vi "Compute Residuals Absolute Area.vi"(8 "Error In":errorcluster, 11 "Residual Plot in":cluster{"X Array":dbl[], "Y Array":dbl[]}) -> (0 "Error Out":errorcluster, 2 "Residuals Area":dbl, 4 "Message":string)   [LabVIEW 2021, in "Fits.lvlib"]
uses:
  Fits.lvlib
  96a839f7-c8a8-4ca7-9598-f59a8eb3621a.vi
panel:
  # "see the License on the block diagram (Ctrl+E or Window:Show Block Diagram)"
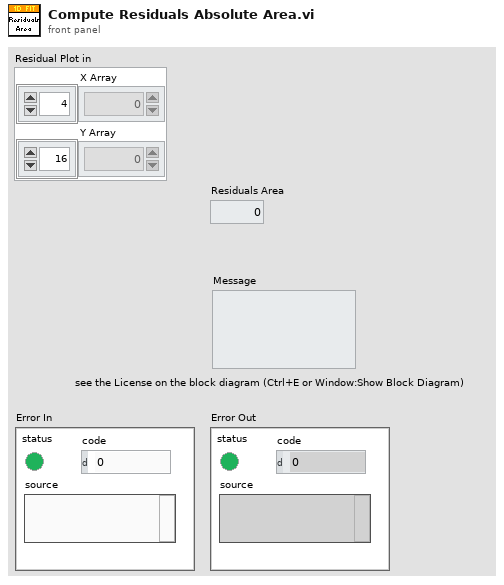
[diagram p1: front panel]
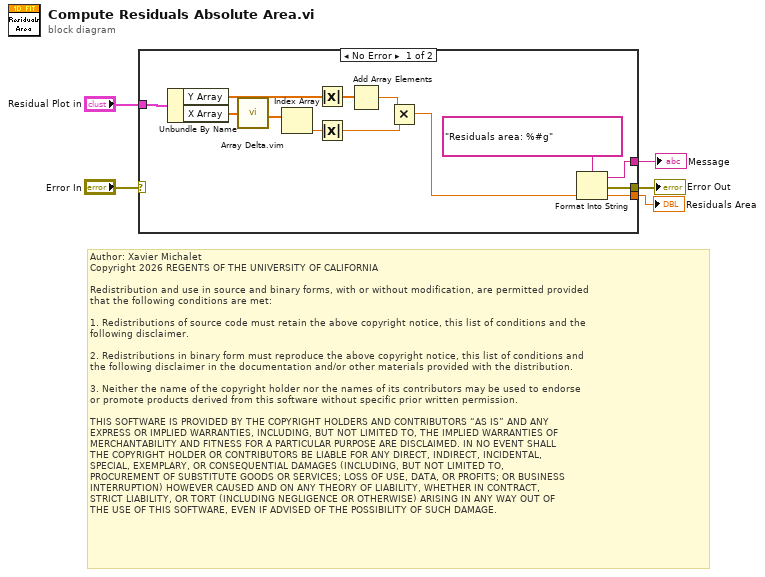
[diagram p0: block diagram]
diagram:
  # "Author: Xavier Michalet\nCopyright 2026 REGENTS OF THE UNIVERSITY OF CALIFORNIA\n\nRedistribution and use in source and binary forms, with or without modification, are permitted provided\nthat the following conditions are met:\n\n1. Redistributions of source code must retain the above copyright notice, this list of conditions and the\nfollowing disclaimer.\n\n2. Redistributions in binary form must reproduce the above copyright notice, this list of conditions and\nthe following disclaimer in the documentation and/or other materials provided with the distribution.\n\n3. Neither the name of the copyright holder nor the names of its contributors may be used to endorse \nor promote products derived from this software without specific prior written permission.\n\nTHIS SOFTWARE IS PROVIDED BY THE COPYRIGHT HOLDERS AND CONTRIBUTORS “AS IS” AND ANY \nEXPRESS OR IMPLIED WARRANTIES, INCLUDING, BUT NOT LIMITED TO, THE IMPLIED WARRANTIES OF\nMERCHANTABILITY AND FITNESS FOR A PARTICULAR PURPOSE ARE DISCLAIMED. IN NO EVENT SHALL\nTHE COPYRIGHT HOLDER OR CONTRIBUTORS BE LIABLE FOR ANY DIRECT, INDIRECT, INCIDENTAL, \nSPECIAL, EXEMPLARY, OR CONSEQUENTIAL DAMAGES (INCLUDING, BUT NOT LIMITED TO, \nPROCUREMENT OF SUBSTITUTE GOODS OR SERVICES; LOSS OF USE, DATA, OR PROFITS; OR BUSINESS\nINTERRUPTION) HOWEVER CAUSED AND ON ANY THEORY OF LIABILITY, WHETHER IN CONTRACT, \nSTRICT LIABILITY, OR TORT (INCLUDING NEGLIGENCE OR OTHERWISE) ARISING IN ANY WAY OUT OF\nTHE USE OF THIS SOFTWARE, EVEN IF ADVISED OF THE POSSIBILITY OF SUCH DAMAGE."
  n1 = case shown="No Error" "Error In" {
    selector: "Error In" -> [_ w18]
    tunnel: [w16 w18] -> w4
    tunnel: "Residual Plot in" -> [w17 _]
    tunnel: [w14 _] -> w2
    tunnel: [w6 _] -> w1
    frame No Error {
      n2 = Unbundle By Name(w17) -> ("Y Array"=w13:dbl[], "X Array"=w12:dbl[])
      n3 = call "Array Delta.vim"("A"=w12) -> ("A[i+1]-A[i]"=w11:dbl[])  [unwired: 8 in]
      n4 = Index Array(array=w11) -> (element=w10:dbl)  [unwired: 1 in]
      n5 = Absolute Value(x=w13) -> (abs(x)=w9:dbl[])
      n6 = Absolute Value(x=w10) -> (abs(x)=w7:dbl)
      n7 = Add Array Elements(numeric array=w9) -> (sum=w8:dbl)
      n8 = Multiply(x=w8, y=w7) -> (x*y=w6:dbl)
      n9 = Format Into String(format string="Residuals area: %#g", w6) -> (resulting string=w14:string, error out=w16:errorcluster)  [unwired: 2 in]
    }
    frame Error {
    }
  }
  "Error Out" <- w4
  "Message" <- w2
  "Residuals Area" <- w1
